vi "Control TransAO.vi"(0 "VISA resource name":refnum<visa-resource-name>, 5 "All or Spcified channels (All)":bool=TRUE, 7 "Selected All channels":cluster{"Transfer output (On) ":bool}={"Transfer output (On) "=TRUE}, 9 "Selected Specified channels":cluster{"Channels (0001-On)":string}={"Channels (0001-On)"="0001-On"}, 11 "error in":errorcluster) -> (4 "VISA resource name out":refnum<visa-resource-name>, 15 "error out":errorcluster)   [LabVIEW 2020, in "Yokogawa GX Series.lvlib"]
doc: "Control transfer output of AO channel."
uses:
  <instrlib>/Yokogawa GX Series/Yokogawa GX Series.lvlib
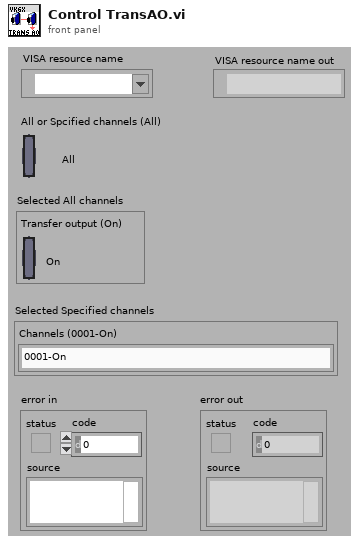
[diagram p1: front panel]
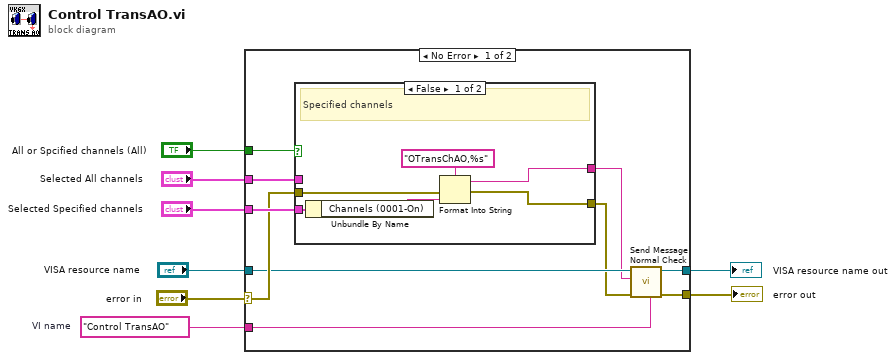
[diagram p0: block diagram]
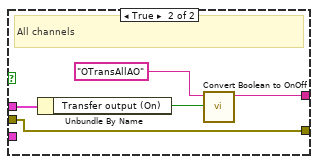
[diagram p2: hidden frame]
diagram:
  w4 = "Control TransAO"  # VI name
  n1 = case shown="No Error" "error in" {
    selector: "error in" -> [w13 w31]
    tunnel: [w18 w30] -> w1
    tunnel: [w17 w31] -> w2
    tunnel: "All or Spcified channels (All)" -> [w16 _]
    tunnel: "Selected All channels" -> [w15 _]
    tunnel: "Selected Specified channels" -> [w14 _]
    tunnel: w4 -> [w12 _]
    tunnel: "VISA resource name" -> [w11 w30]
    frame No Error {
      n2 = case shown="False" w16 {
        tunnel: w15 -> [_ w27]
        tunnel: w14 -> [w23 _]
        tunnel: w13 -> [w21 w25]
        tunnel: [w20 w26] -> w9
        tunnel: [w19 w25] -> w10
        frame False {
          # "Specified channels"
          n3 = Unbundle By Name(w23) -> ("Channels (0001-On)"=w22:string)
          n4 = Format Into String(format string="OTransChAO,%s", error in=w21, w22) -> (resulting string=w20:string, error out=w19:errorcluster)  [unwired: 1 in]
        }
        frame True {
          # "All channels"
          n5 = Unbundle By Name(w27) -> ("Transfer output (On)"=w29:bool)
          n6 = call <instrlib>:"Convert Boolean to OnOff.vi"("On/Off"=w29, "Initial String (\"\")"="OTransAllAO") -> ("Resulting String"=w26:string)  [unwired: 9 in]
        }
      }
      n7 = call <instrlib>:"Send Message Normal Check.vi"("Source (\"\")"=w12, "error in (no error)"=w10, "Send Message (\"\")"=w9, "VISA resource name"=w11) -> ("error out"=w17:errorcluster, "VISA resource name out"=w18:refnum<visa-resource-name>)  [unwired: 2 in, 4 out]
    }
    frame Error {
    }
  }
  "VISA resource name out" <- w1
  "error out" <- w2
